vi "Calculate merit factor.vi"(8 "error in (no error)":errorcluster, 11 "DAQOrcaFlash in":refnum<class "DAQOrcaFlash.lvclass">) -> (0 "error out":errorcluster, 3 "DAQOrcaFlash out":refnum<class "DAQOrcaFlash.lvclass">)   [LabVIEW 2012, in "DAQOrcaFlash.lvclass"]
uses:
  DAQOrcaFlash.lvclass
  DAQOrcaFlash.lvclass/DAQOrcaFlash.ctl
  <vilib>/Analysis/baseanly.llb/Mean (DBL).vi
  <vilib>/Analysis/NI_AALBase.lvlib
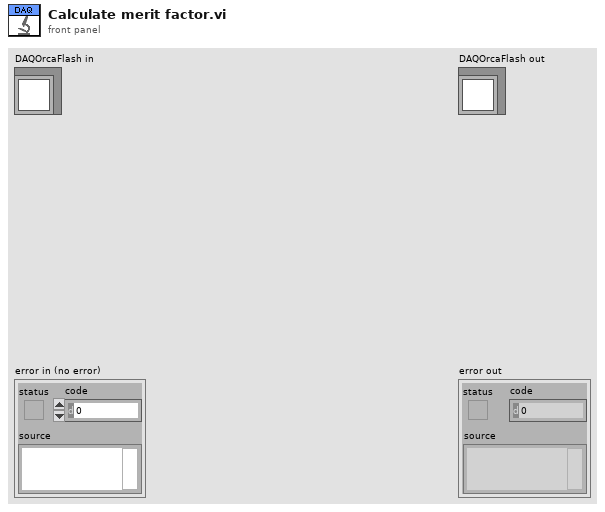
[diagram p1: front panel]
types:
  T1 = typedef "DAQOrcaFlash.lvclass/merit_factor_type.ctl" = enum16{"full frame intensity", "5% brightest"}
  T2 = typedef "IMAQ Image.ctl" = refnum<image>
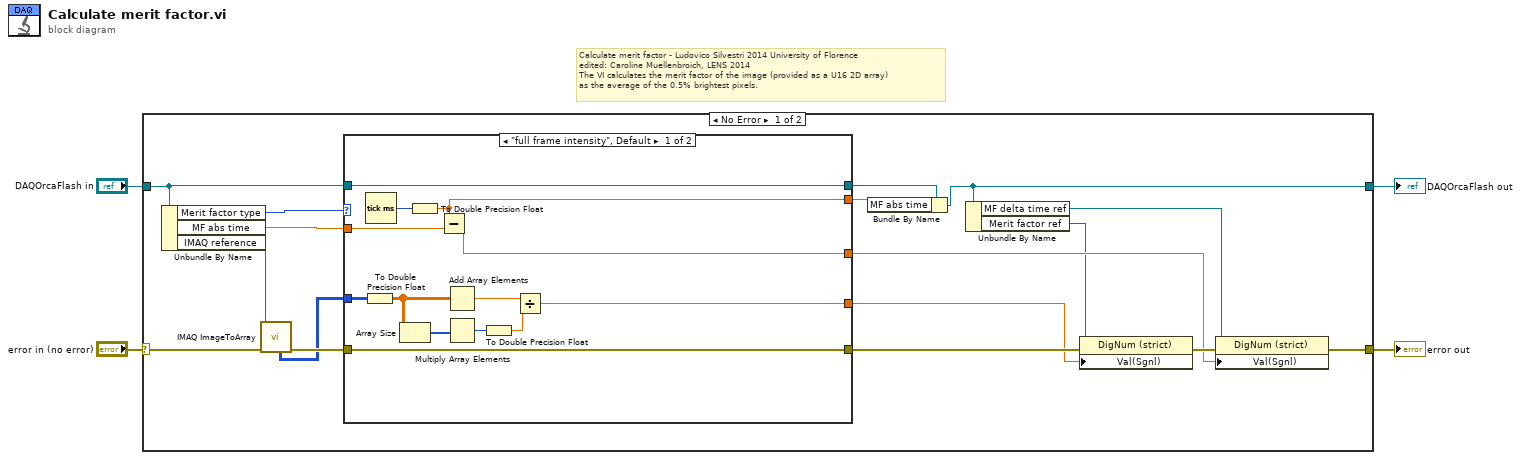
[diagram p0: block diagram]
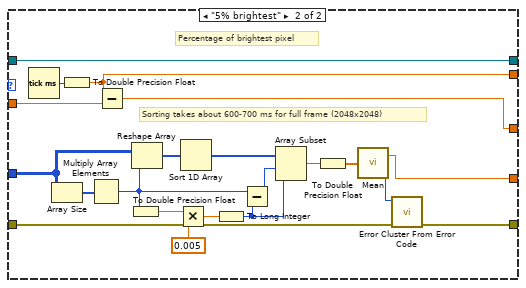
[diagram p2: hidden frame]
diagram:
  # "Calculate merit factor - Ludovico Silvestri 2014 University of Florence\nedited: Caroline Muellenbroich, LENS 2014\nThe VI calculates the merit factor of the image (provided as a U16 2D array)\nas the average of the 0.5% brightest pixels."
  n1 = case shown="No Error" "error in (no error)" {
    selector: "error in (no error)" -> [w7 w56]
    tunnel: [w12 w56] -> w4
    tunnel: "DAQOrcaFlash in" -> [w19 w57]
    tunnel: [w14 w57] -> w2
    frame No Error {
      n2 = Unbundle By Name(w19) -> ("Merit factor type"=w20:T1, "MF abs time"=w18:dbl, "IMAQ reference"=w8:T2)
      n3 = call "IMAQ ImageToArray"("error in (no error)"=w7, "Image"=w8) -> ("Image Pixels (U16)"=w5:u16[][], "error out"=w6:errorcluster)  [unwired: 2 in, 3 out]
      n4 = case shown="\"full frame intensity\", Default" w20 {
        tunnel: [w34 w54] -> w21
        tunnel: w6 -> [w34 w42]
        tunnel: w5 -> [w33 w41]
        tunnel: w19 -> [w29 w40]
        tunnel: [w29 w40] -> w15
        tunnel: w18 -> [w32 w39]
        tunnel: [w31 w38] -> w11
        tunnel: [w22 w37] -> w17
        tunnel: [w28 w36] -> w16
        frame "full frame intensity", Default {
          n5 = To Double Precision Float(number=w33) -> (double precision float=w26:dbl[][])
          n6 = Tick Count (ms)() -> (millisecond timer value=w30:u32)
          n7 = Array Size(array=w26) -> (size(s)=w25:i32[])
          n8 = To Double Precision Float(number=w30) -> (double precision float=w28:dbl)
          n9 = Subtract(x=w28, y=w32) -> (x-y=w31:dbl)
          n10 = Add Array Elements(numeric array=w26) -> (sum=w27:dbl)
          n11 = Multiply Array Elements(1:w25) -> (0:w24:i32)
          n12 = To Double Precision Float(number=w24) -> (double precision float=w23:dbl)
          n13 = Divide(x=w27, y=w23) -> (x/y=w22:dbl)
        }
        frame "5% brightest" {
          # "Percentage of brightest pixel"
          # "Sorting takes about 600-700 ms for full frame (2048x2048)"
          n14 = Tick Count (ms)() -> (millisecond timer value=w35:u32)
          n15 = Array Size(array=w41) -> (size(s)=w50:i32[])
          n16 = To Double Precision Float(number=w35) -> (double precision float=w36:dbl)
          n17 = Multiply Array Elements(1:w50) -> (0:w43:i32)
          n18 = Subtract(x=w36, y=w39) -> (x-y=w38:dbl)
          n19 = To Double Precision Float(number=w43) -> (double precision float=w49:dbl)
          n20 = Reshape Array(w41, w43) -> (w51:u16[])
          n21 = Multiply(x=w49, y=0.005) -> (x*y=w47:dbl)
          n22 = Sort 1D Array(array=w51) -> (sorted array=w52:u16[])
          n23 = To Long Integer(number=w47) -> (32bit integer=w46:i32)
          n24 = Subtract(x=w43, y=w46) -> (x-y=w45:i32)
          n25 = Array Subset(array=w52, index=w45, length=w46) -> (w44:u16[])
          n26 = To Double Precision Float(number=w44) -> (double precision float=w53:dbl[])
          n27 = call-poly <vilib>:"Mean.vi"("X"=w53) -> ("mean"=w37:dbl, "error"=w55:i32)
          n28 = call <vilib>:"Error Cluster From Error Code.vi"("error in (no error)"=w42, "error code (0)"=w55) -> ("error out"=w54:errorcluster)  [unwired: 7 in]
        }
      }
      n29 = Bundle By Name(cluster=w15, "MF abs time"=w16) -> (w14:refnum<class "DAQOrcaFlash.lvclass">)
      n30 = Unbundle By Name(w14) -> ("MF delta time ref"=w9:refnum<vi>, "Merit factor ref"=w10:refnum<vi>)
      n31 = property class="DigNum (strict)"(reference=w10, error in=w21, "Val(Sgnl)"=w17) -> (error out=w13:errorcluster)  [unwired: 1 out]
      n32 = property class="DigNum (strict)"(reference=w9, error in=w13, "Val(Sgnl)"=w11) -> (error out=w12:errorcluster)  [unwired: 1 out]
    }
    frame Error {
    }
  }
  "error out" <- w4
  "DAQOrcaFlash out" <- w2
